vi "Get Chemistries.vi"(0 "reference in":refnum<class "Battery.lvclass">, 5 "Error In":errorcluster) -> (14 "reference out":refnum<class "Battery.lvclass">, 16 "chemistries":string[](array[string]), 19 "Error Out":errorcluster)   [LabVIEW 2023, in "Battery.lvclass"]
uses:
  Battery.lvclass
  Battery.lvclass/Battery.ctl
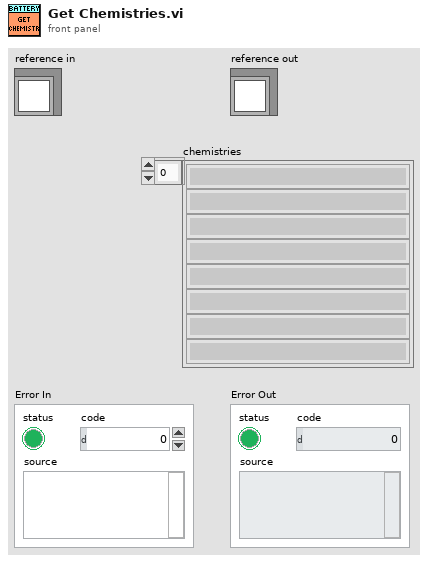
[diagram p1: front panel]
types:
  T1 = typedef "Battery.lvclass/ObjectAttributes.ctl" = cluster{"Python module":path, "Python Session":refnum<k35>, "PybammWrapper":refnum<k38>, "Cell Voltage (V)":dbl, "Cell Current (A)":dbl, "SoC (%)":dbl}
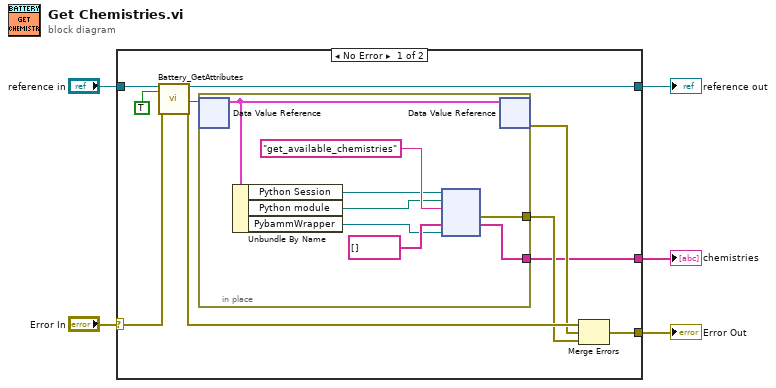
[diagram p0: block diagram]
diagram:
  n1 = case shown="No Error" "Error In" {
    selector: "Error In" -> [w14 w25]
    tunnel: [w12 w25] -> w4
    tunnel: [w13 w24] -> w2
    tunnel: "reference in" -> [w15 w24]
    tunnel: [w6 _] -> w1
    frame No Error {
      n2 = call "Battery_GetAttributes.vi"("reference in"=w15, "OnlyGetDvrReference(False)"=TRUE, "Error In"=w14) -> ("reference out"=w13:refnum<class "Battery.lvclass">, "DataRef"=w11:refnum<data-value>, "Error Out"=w9:errorcluster)  [unwired: 13 in, 1 out]
      n3 = in-place {
        in-place-border: [w17] -> w7
        in-place-border: [w16] -> w6
        n4 = in-place-dvr #1(w11) -> (w23:T1)  [unwired: 1 out]
        n5 = Unbundle By Name(w23) -> ("Python Session"=w19:refnum<k35>, "Python module"=w18:path, "PybammWrapper"=w20:refnum<k38>)
        n6 = node(w19, w18, "get_available_chemistries" ("function name"), string[] [], w20) -> (w17:errorcluster, w16:string[])  [unwired: 2 in, 3 out]
        n7 = in-place-dvr #1(w23) -> (w8:errorcluster)  [unwired: 1 out]
      }
      n8 = Merge Errors(w9, w8, w7) -> (w12:errorcluster)
    }
    frame Error {
    }
  }
  "Error Out" <- w4
  "reference out" <- w2
  "chemistries" <- w1
